vi "Save.vi"(8 "error in (no error)":errorcluster, 9 "File name":string, 10 "Inpath":path, 11 "CNN in":refnum<class "CNN.lvclass">) -> (0 "error out":errorcluster, 3 "CNN out":refnum<class "CNN.lvclass">)   [LabVIEW 2016, in "CNN.lvclass"]
uses:
  CNN.lvclass
  <vilib>/Utility/xml.llb/Write to XML File(string).vi
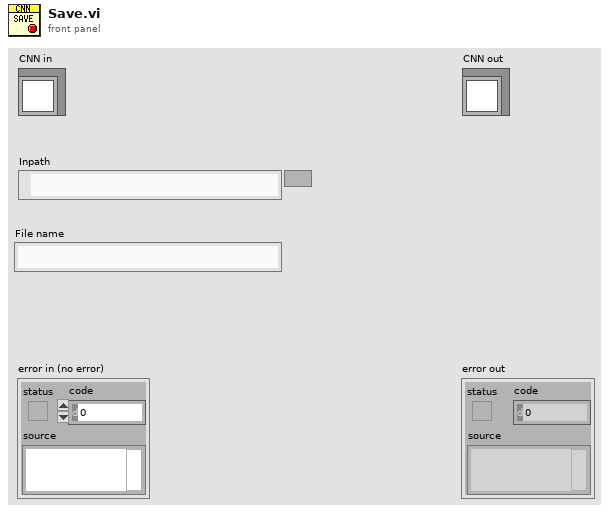
[diagram p1: front panel]
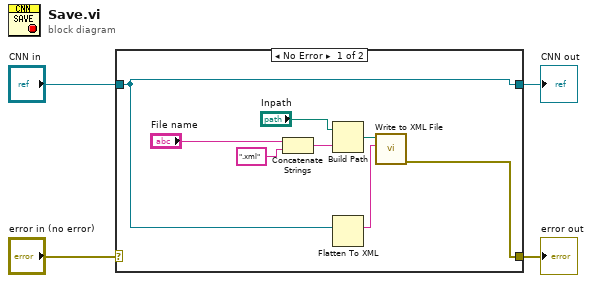
[diagram p0: block diagram]
diagram:
  n1 = case shown="No Error" "error in (no error)" {
    selector: "error in (no error)" -> [_ w13]
    tunnel: [w5 w13] -> w3
    tunnel: [w6 w14] -> w1
    tunnel: "CNN in" -> [w6 w14]
    frame No Error {
      n2 = Concatenate Strings("File name", ".xml" ("name or relative path")) -> (w9:string)
      n3 = Build Path(base path="Inpath", name or relative path=w9) -> (appended path=w11:path)
      n4 = Flatten To XML(anything=w6) -> (xml string=w12:string)
      n5 = call-poly <vilib>:"Write to XML File.vi"("XML Input"=w12, "XML File Path"=w11) -> ("error out"=w5:errorcluster)  [unwired: 7 in, 2 out]
    }
    frame Error {
    }
  }
  "error out" <- w3
  "CNN out" <- w1
